vi "Analysis.Filter Result Summaries.vi"(10 "Filters":T2 {"Date2" items=["2019-01-01"]; "Date1" items=["2019-01-01"]}, 11 "ResultSum":T1[](array[typedef])) -> (3 "Filtered ResultSum":T1[](array[typedef]))   [LabVIEW 2024]
uses:
  Analysis.Result Summary Filters.ctl
  Analysis.Result Summary.ctl
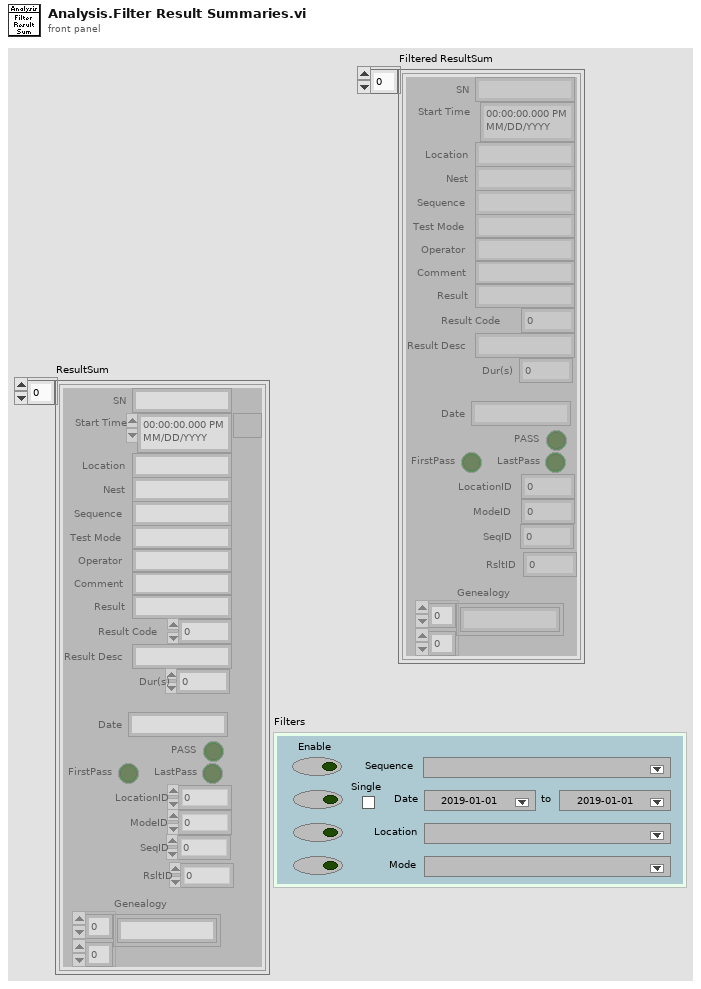
[diagram p1: front panel]
types:
  T1 = typedef "Analysis.Result Summary.ctl" = cluster{"SN":string, "Start Time":timestamp, "Location":string, "Nest":string, "Sequence":string, "Operator":string, "Test Mode":string, "Comment":string, "Result":string, "Result Code":i32, "Result Desc":string, "Date":string, "Dur(s)":dbl, "PASS":bool, "FirstPass":bool, "LastPass":bool, "LocationID":i32, "ModeID":i32, "SeqID":i32, "RsltID":i32, "Genealogy":string[][]}
  T2 = typedef "Analysis.Result Summary Filters.ctl" = cluster{"Filter En Seq":bool, "Sequence":u16, "Filter En Date":bool, "Date1":u16, "Location":u16, "Filter En Loc":bool, "Mode":u16, "Filter En Mode":bool, "Seq List":string[], "Date List":string[], "Loc List":string[], "Mode List":string[], "Date2":u16, "Date Range":bool}
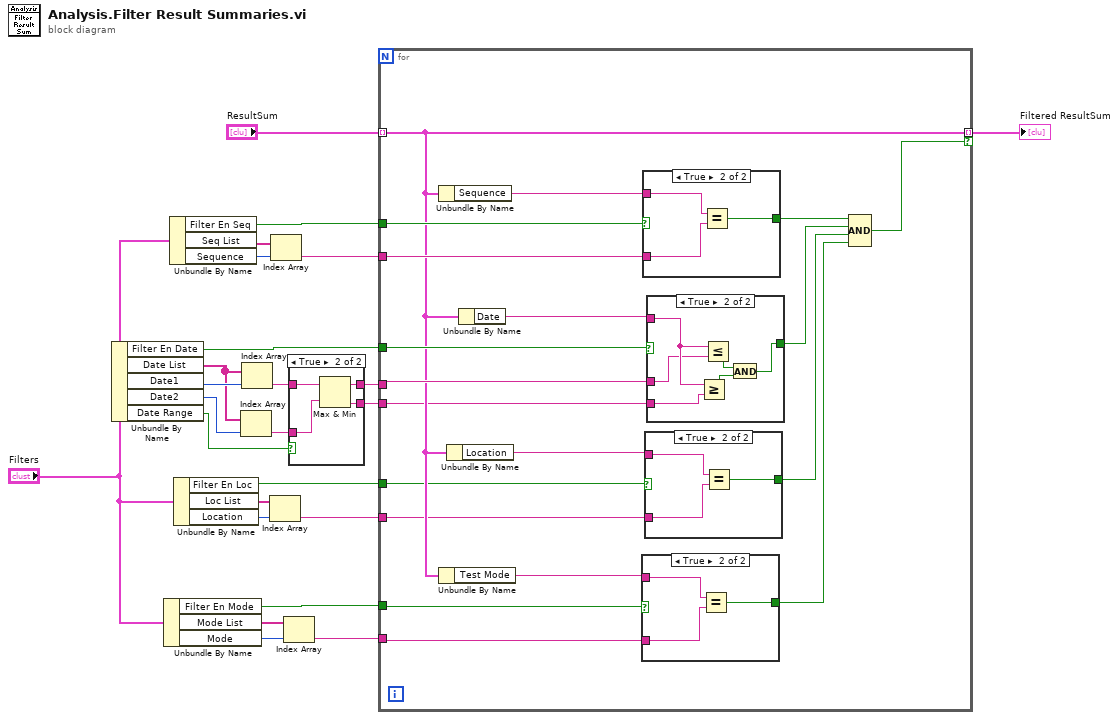
[diagram p0: block diagram]
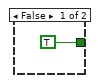
[diagram p3: hidden frame]
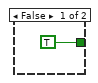
[diagram p4: hidden frame]
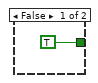
[diagram p5: hidden frame]
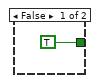
[diagram p6: hidden frame]
diagram:
  n1 = Unbundle By Name("Filters") -> ("Filter En Date"=w21:bool, "Date List"=w7:string[], "Date1"=w22:u16, "Date2"=w6:u16, "Date Range"=w1:bool)
  n2 = Unbundle By Name("Filters") -> ("Filter En Mode"=w10:bool, "Mode List"=w15:string[], "Mode"=w14:u16)
  n3 = Unbundle By Name("Filters") -> ("Filter En Seq"=w17:bool, "Seq List"=w19:string[], "Sequence"=w20:u16)
  n4 = Unbundle By Name("Filters") -> ("Filter En Loc"=w9:bool, "Loc List"=w16:string[], "Location"=w13:u16)
  n5 = Index Array(array=w7, index=w6) -> (element=w4:string)
  n6 = Index Array(array=w7, index=w22) -> (element=w5:string)
  n7 = Index Array(array=w16, index=w13) -> (element=w12:string)
  n8 = Index Array(array=w19, index=w20) -> (element=w18:string)
  n9 = Index Array(array=w15, index=w14) -> (element=w11:string)
  n10 = case shown="True" w1 {
    tunnel: w5 -> [w25 w29]
    tunnel: w4 -> [_ w28]
    tunnel: [w25 w27] -> w3
    tunnel: [w25 w26] -> w2
    frame False {
    }
    frame True {
      n11 = Max & Min(x=w29, y=w28) -> (max(x,y)=w27:string, min(x,y)=w26:string)
    }
  }
  n12 = for {
    tunnel: "ResultSum" -> [w39] mode=indexing
    tunnel: [w39] -> w23 mode=indexing if=w31
    tunnel: w21 -> [w43]
    tunnel: w3 -> [w42]
    tunnel: w18 -> [w46]
    tunnel: w17 -> [w47]
    tunnel: w12 -> [w35]
    tunnel: w11 -> [w36]
    tunnel: w10 -> [w38]
    tunnel: w9 -> [w37]
    tunnel: w2 -> [w30]
    n13 = Unbundle By Name(w39) -> ("Sequence"=w48:string)
    n14 = Unbundle By Name(w39) -> ("Test Mode"=w40:string)
    n15 = Unbundle By Name(w39) -> ("Location"=w41:string)
    n16 = Unbundle By Name(w39) -> ("Date"=w44:string)
    n17 = case shown="True" w38 {
      tunnel: w40 -> [_ w52]
      tunnel: w36 -> [_ w51]
      tunnel: [TRUE w50] -> w32
      frame False {
      }
      frame True {
        n18 = Equal?(x=w52, y=w51) -> (x = y?=w50:bool)
      }
    }
    n19 = case shown="True" w47 {
      tunnel: w48 -> [_ w67]
      tunnel: w46 -> [_ w66]
      tunnel: [TRUE w65] -> w45
      frame False {
      }
      frame True {
        n20 = Equal?(x=w67, y=w66) -> (x = y?=w65:bool)
      }
    }
    n21 = case shown="True" w37 {
      tunnel: w41 -> [_ w56]
      tunnel: w35 -> [_ w55]
      tunnel: [TRUE w54] -> w33
      frame False {
      }
      frame True {
        n22 = Equal?(x=w56, y=w55) -> (x = y?=w54:bool)
      }
    }
    n23 = case shown="True" w43 {
      tunnel: w44 -> [_ w59]
      tunnel: w42 -> [_ w58]
      tunnel: [TRUE w61] -> w34
      tunnel: w30 -> [_ w63]
      frame False {
      }
      frame True {
        n24 = Greater Or Equal?(x=w59, y=w63) -> (x >= y?=w62:bool)
        n25 = Less Or Equal?(x=w59, y=w58) -> (x <= y?=w60:bool)
        n26 = And(x=w60, y=w62) -> (x .and. y?=w61:bool)
      }
    }
    n27 = Compound Arithmetic op=AND(w45, w34, w33, w32) -> (w31:bool)
  }
  "Filtered ResultSum" <- w23
